vi "test CAN Cyclic Loopback with Information Channels.vi"(8 "error in (no error)":errorcluster, 11 "TestCase in":refnum<class "CAN Loopback Tests.lvclass">) -> (0 "error out":errorcluster, 3 "TestCase out":refnum<class "CAN Loopback Tests.lvclass">)   [LabVIEW 2017, in "CAN Loopback Tests.lvclass"]
uses:
  CAN Loopback Tests.lvclass
  <vilib>/addons/_JKI Toolkits/VI Tester/TestCase.llb/TestCase.lvclass
  C:/Program Files (x86)/National Instruments/LabVIEW 2017/vi.lib/addons/_JKI Toolkits/VI Tester/TestCase.llb/TestCase.lvclass
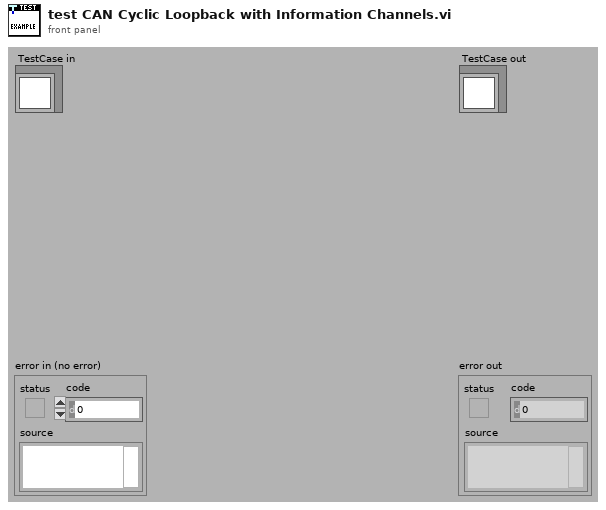
[diagram p1: front panel]
types:
  T1 = cluster{"loopback channels to write":string[], "loopback channels to read":string[], "additional channels to write":string[], "additional channels to read":string[]}
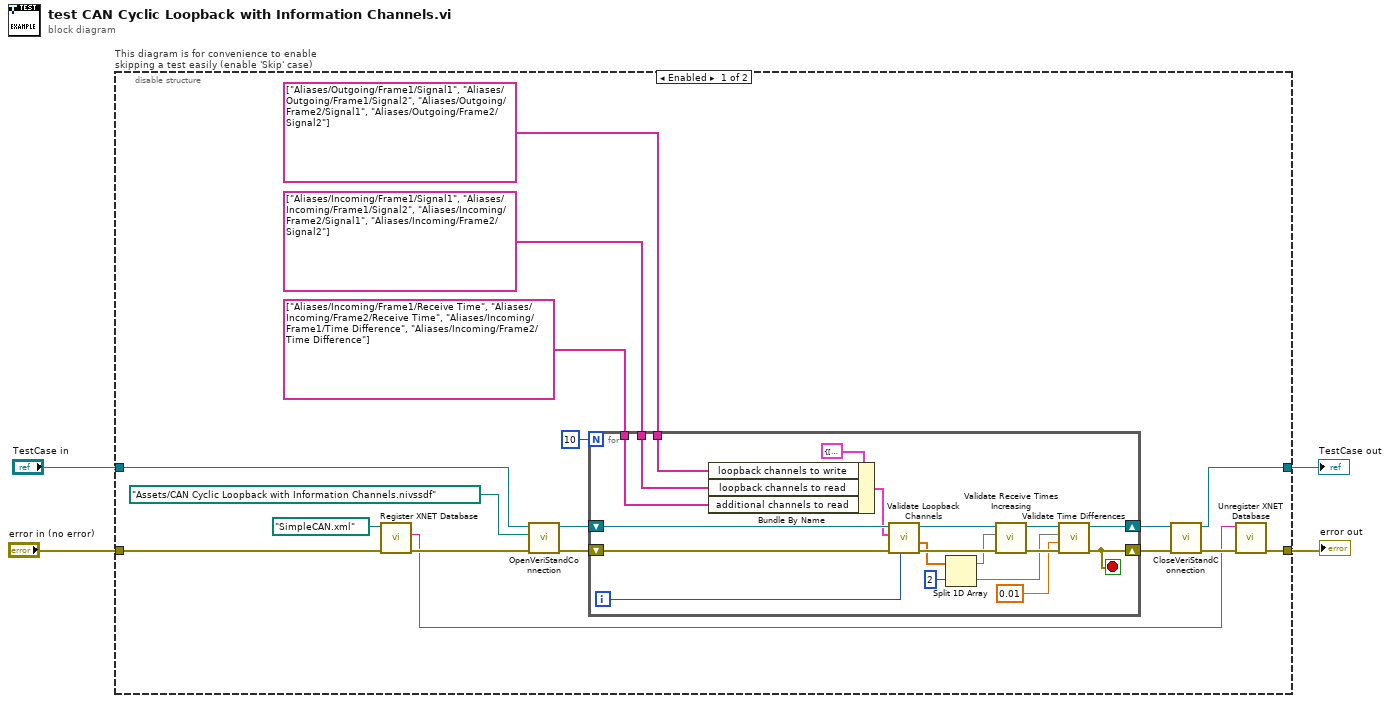
[diagram p0: block diagram]
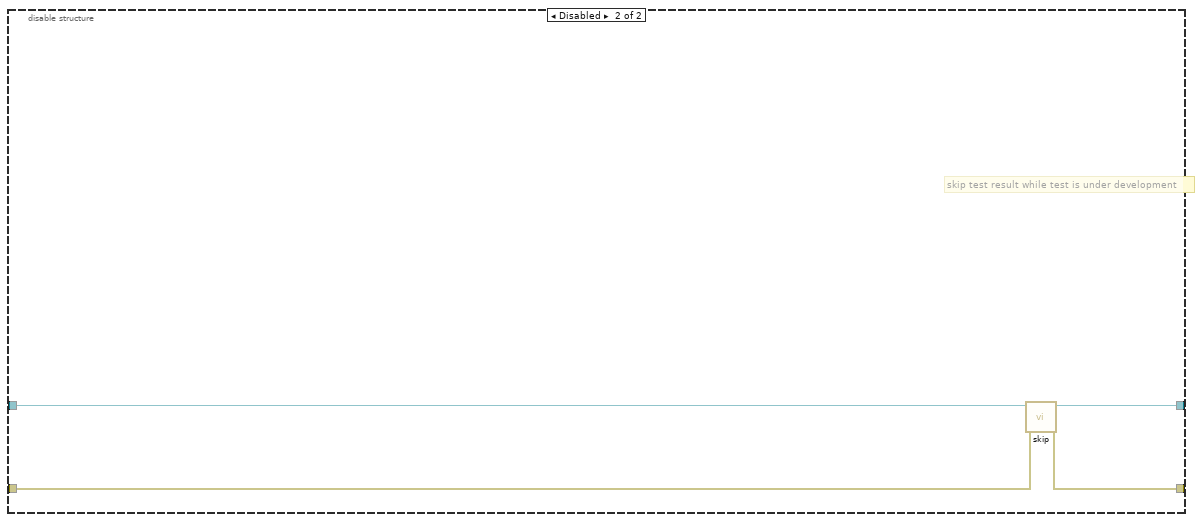
[diagram p2: hidden frame]
diagram:
  n1 = disable-structure "This diagram is for convenience to enable skipping a test easily (enable 'Skip' case)" shown="Enabled" {
    disable-tunnel: "TestCase in" -> [w21 w44]
    disable-tunnel: [w18 w42] -> w1
    disable-tunnel: [w9 w43] -> w3
    disable-tunnel: "error in (no error)" -> [w11 w41]
    frame Enabled {
      n2 = call "Register XNET Database.vi"("error in (no error)"=w11, "database path"=path "SimpleCAN.xml") -> ("error out"=w10:errorcluster, "alias"=w7:string)  [unwired: 8 in]
      n3 = call-dynamic "OpenVeriStandConnection.vi"("error in (no error)"=w10, "System Definition File"=path "Assets/CAN Cyclic Loopback with Information Channels.nivssdf", "VeriStand Test Case in"=w21) -> ("error out"=w19:errorcluster, "VeriStand Test Case out"=w5:refnum<class "CAN Loopback Tests.lvclass">)  [unwired: 6 in, 1 out]
      n4 = for {
        N: 10 -> [_]
        shift-right: [w34] -> w16
        shift-left: w19 -> [w40]
        shift-right: [w33] -> w17
        shift-left: w5 -> [w39]
        tunnel: string[] ["Aliases/Incoming/Frame1/Signal1", "Aliases/Incoming/Frame1/Signal2", "Aliases/Incoming/Frame2/Signal1", "Aliases/Incoming/Frame2/Signal2"] -> [w30]
        tunnel: string[] ["Aliases/Outgoing/Frame1/Signal1", "Aliases/Outgoing/Frame1/Signal2", "Aliases/Outgoing/Frame2/Signal1", "Aliases/Outgoing/Frame2/Signal2"] -> [w31]
        tunnel: string[] ["Aliases/Incoming/Frame1/Receive Time", "Aliases/Incoming/Frame2/Receive Time", "Aliases/Incoming/Frame1/Time Difference", "Aliases/Incoming/Frame2/Time Difference"] -> [w29]
        i -> [w23]
        stop <- w34 stop-if-true
        n5 = Bundle By Name(cluster=T1 {"loopback channels to write"=[], "loopback channels to read"=[], "additional channels to write"=[], "additional channels to read"=[]} ("channels"), "loopback channels to write"=w31, "loopback channels to read"=w30, "additional channels to read"=w29) -> (w32:T1)
        n6 = call "Validate Loopback Channels.vi"("index"=w23, "error in (no error)"=w40, "channels"=w32, "CAN Loopback Tests in"=w39) -> ("error out"=w38:errorcluster, "additional channel values to read"=w22:dbl[], "CAN Loopback Tests out"=w37:refnum<class "CAN Loopback Tests.lvclass">)  [unwired: 4 in, 1 out]
        n7 = Split 1D Array(array=w22, index=2) -> (first subarray=w27:dbl[], second subarray=w26:dbl[])
        n8 = call "Validate Receive Times Increasing.vi"("error in (no error)"=w38, "receive times"=w27, "CAN Loopback Tests in"=w37) -> ("error out"=w35:errorcluster, "CAN Loopback Tests out"=w36:refnum<class "CAN Loopback Tests.lvclass">)  [unwired: 7 in]
        n9 = call "Validate Time Differences.vi"("error in (no error)"=w35, "expected value"=0.01, "time differences"=w26, "CAN Loopback Tests in"=w36) -> ("error out"=w34:errorcluster, "CAN Loopback Tests out"=w33:refnum<class "CAN Loopback Tests.lvclass">)  [unwired: 6 in]
      }
      n10 = call-dynamic "CloseVeriStandConnection.vi"("error in (no error)"=w16, "VeriStand Test Case in"=w17) -> ("error out"=w8:errorcluster, "VeriStand Test Case out"=w18:refnum<class "CAN Loopback Tests.lvclass">)  [unwired: 8 in]
      n11 = call "Unregister XNET Database.vi"("error in (no error)"=w8, "alias"=w7) -> ("error out"=w9:errorcluster)  [unwired: 9 in]
    }
    frame Disabled {
      # "skip test result while test is under development"
      n12 = call <vilib>:"skip.vi"("error in (no error)"=w41, "TestCase in"=w44) -> ("error out"=w43:errorcluster, "TestCase out"=w42:refnum<class "CAN Loopback Tests.lvclass">)  [unwired: 8 in]
    }
  }
  "error out" <- w3
  "TestCase out" <- w1
